vi "Reset Engine.vi"(8 "error in (no error)":errorcluster, 11 "Abstract Engine":refnum<class "Abstract Engine.lvclass">) -> (0 "error out":errorcluster, 3 "Abstract Engine out":refnum<class "Abstract Engine.lvclass">)   [LabVIEW 2025, in "Abstract Engine.lvlib" / "Abstract Engine.lvclass"]
uses:
  Abstract Engine.lvclass
  C:/Users/Public/Documents/Sandia National Labs/TSS Plugin/CEF.lvlibp/Node/CEF_Node.lvclass
  Engine configuration/Engine configuration.lvclass
  Engine Cluster.ctl
  Abstract Instrument/Channel.ctl
  Engine configuration/Engine configuration.lvclass/Engine configuration.ctl
  Abstract Engine.lvclass/Abstract Engine.ctl
  Abstract Instrument/Abstract Instrument.lvclass
  Engine configuration/Read Engine Setting.vi
  Write Engine Cluster.vi
  Users/Public/Documents/Sandia National Labs/TSS Plugin/CEF.lvlibp/Node/ReadChildren.vi
  Users/Public/Documents/Sandia National Labs/TSS Plugin/CEF.lvlibp/serializable configuration/CEF_serializable configuration.lvclass
  Users/Public/Documents/Sandia National Labs/TSS Plugin/CEF.lvlibp/Node/CEF_Node.lvclass
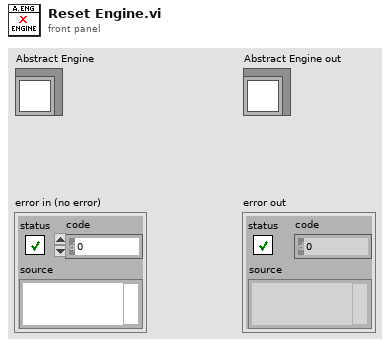
[diagram p1: front panel]
types:
  T1 = typedef "Abstract Engine.lvlib/Abstract Engine.lvclass/Engine Cluster.ctl" = cluster{"IP Address":string, "Type":string, "Initialized":bool, "InstrumentMap":map{string, cluster{"Initialized":bool, "Channels":T2[]}}}
  T2 = typedef "Abstract Engine.lvlib/Abstract Instrument.lvclass/Channel.ctl" = cluster{"Alias":string, "DataType":enum16{"Anaolg Input", "Waveform"}, "Unit":enum16{"---", "V", "A", "Ohm", "Hz", "uF", "degC", "deg"}, "Upper limit":dbl, "Lower limit":dbl, "Measurement":variant}
  T3 = typedef "Abstract Engine.lvlib/Engine configuration.lvclass/Engine Setting.ctl" = cluster{"Enabled":bool, "IP Address":string, "Port":i32, "Description":string, "Type":string, "Version":string}
  T4 = map{string, cluster{"Initialized":bool, "Channels":T2[]}}
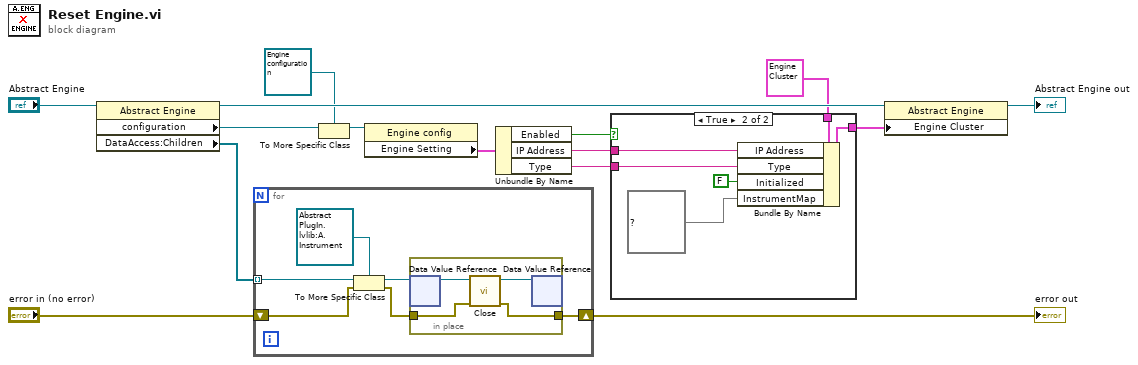
[diagram p0: block diagram]
diagram:
  n1 = property class="Abstract Engine"(reference="Abstract Engine") -> (reference out=w12:refnum<class "Abstract Engine.lvclass">, "configuration"=w5:refnum<class "CEF_serializable configuration.lvclass">, "DataAccess:Children"=w9:refnum<data-value>[])  [unwired: 1 in, 1 out]
  n2 = for {
    tunnel: w9 -> [w21] mode=indexing
    shift-right: [w17] -> w14
    shift-left: "error in (no error)" -> [w19]
    n3 = To More Specific Class(target class=refnum<data-value> refnum ("data value reference"), reference=w21, error in=w19) -> (specific class reference=w20:refnum<data-value>, error out=w18:errorcluster)
    n4 = in-place {
      in-place-border: w18 -> [w23]
      in-place-border: [w22] -> w17
      n5 = in-place-dvr #1(w20) -> (w25:refnum<class "Abstract Instrument.lvclass">)  [unwired: 1 out]
      n6 = call-dynamic "Close.vi"("error in (no error)"=w23, "Abstract Instrument in"=w25) -> ("error out"=w22:errorcluster, "Abstract Instrument out"=w24:refnum<class "Abstract Instrument.lvclass">)  [unwired: 8 in]
      n7 = in-place-dvr #1(w24) -> ()  [unwired: 2 out]
    }
  }
  "error out" <- w14
  n8 = To More Specific Class(target class=refnum<class "Engine configuration.lvclass"> refnum ("Abstract Engine.lvlib:Engine config"), reference=w5) -> (specific class reference=w8:refnum<class "Engine configuration.lvclass">)  [unwired: 1 in, 1 out]
  n9 = property class="Engine config"(reference=w8) -> ("Engine Setting"=w7:T3)  [unwired: 1 in, 2 out]
  n10 = Unbundle By Name(w7) -> ("Enabled"=w4:bool, "IP Address"=w3:string, "Type"=w2:string)
  n11 = case shown="True" w4 {
    tunnel: [w26 w32] -> w10
    tunnel: w3 -> [_ w30]
    tunnel: w2 -> [_ w28]
    tunnel: T1 {"IP Address"="", "Type"="", "Initialized"=FALSE, "InstrumentMap"={}} ("Engine Cluster") -> [w26 w31]
    frame False {
    }
    frame True {
      n12 = Bundle By Name(cluster=w31, "IP Address"=w30, "Type"=w28, "Initialized"=FALSE ("Engine Initialization"), "InstrumentMap"=T4 {}) -> (w32:T1)
    }
  }
  n13 = property class="Abstract Engine"(reference=w12, "Engine Cluster"=w10) -> (reference out=→"Abstract Engine out":refnum<class "Abstract Engine.lvclass">)  [unwired: 1 in, 1 out]
